vi "writeSerialCommunicator.vi"(8 "error in (no error)":errorcluster, 10 "serialCommunicator":refnum<class "SerialCommunicator.lvclass">, 11 "TEI9150 in":refnum<class "TEI9150.lvclass">) -> (0 "error out":errorcluster, 3 "TEI9150 out":refnum<class "TEI9150.lvclass">)   [LabVIEW 2015, in "TEI9150.lvclass"]
uses:
  TEI9150.lvclass
  <userlib>/Common/SerialProtocols/SerialCommunicator/SerialCommunicator.lvclass
  TEI9150.lvclass/TEI9150.ctl
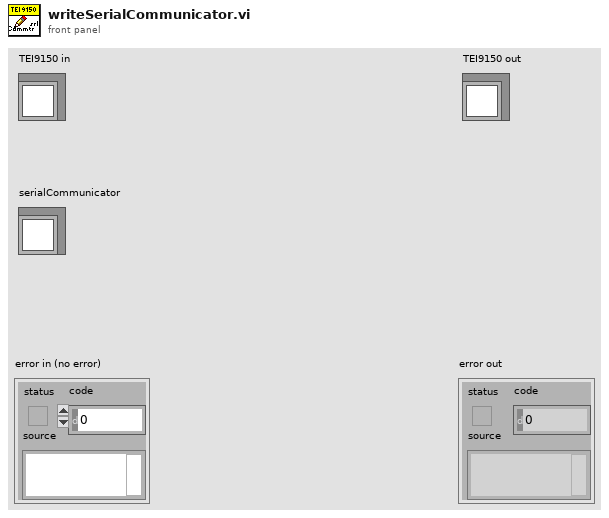
[diagram p1: front panel]
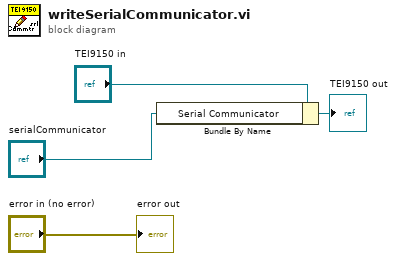
[diagram p0: block diagram]
diagram:
  n1 = Bundle By Name(cluster="TEI9150 in", "Serial Communicator"="serialCommunicator") -> (→"TEI9150 out":refnum<class "TEI9150.lvclass">)
  "error out" <- "error in (no error)"
